vi "test_acupy.vi"() -> ()   [LabVIEW 2023]
uses:
  HoloPyLib/holoTracker.lvlib
panel:
  out "return value":i32
  in  "error in (no error)":errorcluster
  in  "Python version":string="3.10"
  out "error out":errorcluster
  # "Python Node in holoPY.lvlib:HoloPy_test_alloc_CUPY.vi->test_acupy.vi<APPEND>\n\nPython returned the following error: <class 'TypeError'>\n'ndarray' object cannot be interpreted as an integer"
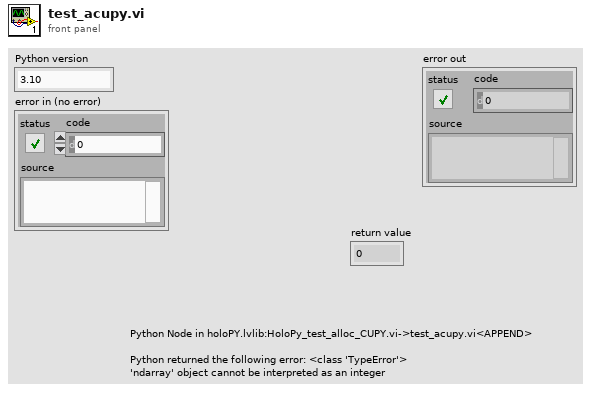
[diagram p1: front panel]
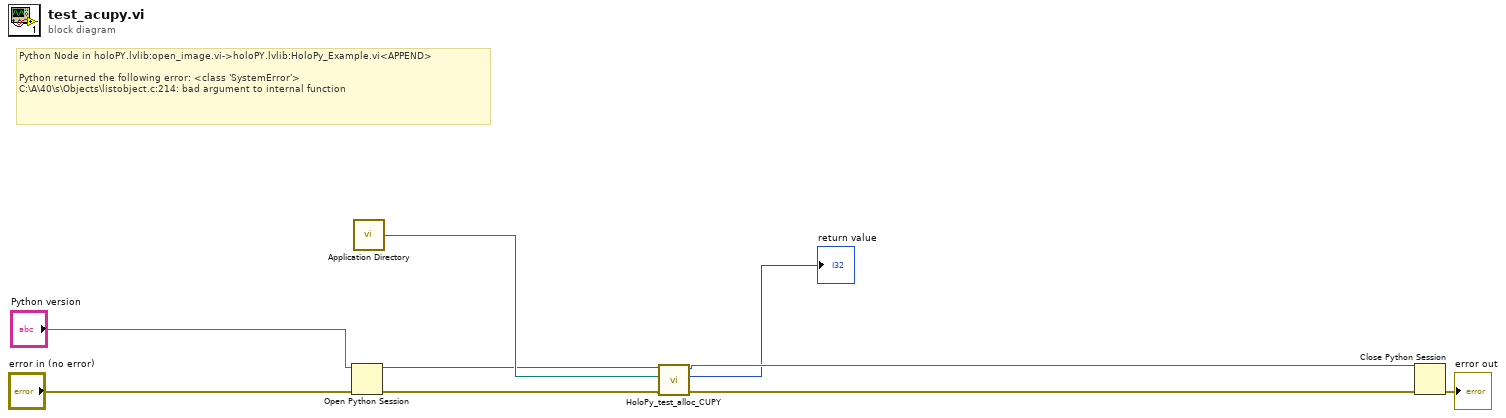
[diagram p0: block diagram]
diagram:
  # "Python Node in holoPY.lvlib:open_image.vi->holoPY.lvlib:HoloPy_Example.vi<APPEND>\n\nPython returned the following error: <class 'SystemError'>\nC:\\A\\40\\s\\Objects\\listobject.c:214: bad argument to internal function"
  n1 = Open Python Session(python version="Python version", 3:"error in (no error)") -> (session out=w4:refnum<k35>, error out=w6:errorcluster)  [unwired: 1 in]
  n2 = call <vilib>:"Application Directory.vi"() -> ("Application Directory"=w5:path)
  n3 = call "HoloPy_test_alloc_CUPY.vi"("error in (no error)"=w6, 10:w5, "Refnum in"=w4) -> ("error out"=w2:errorcluster, "return value"=→"return value":i32, "Refnum out"=w3:refnum<k35>)  [unwired: 6 in]
  n4 = Close Python Session(session in=w3, error in=w2) -> (11:→"error out":errorcluster)
